vi "Set Syntax In Global.vi"(8 "error in":errorcluster, 10 "Syntax":T1, 11 "System no.":i32) -> (0 "error out":errorcluster)   [LabVIEW 2026]
uses:
  Syntax.ctl
  Global1.vi
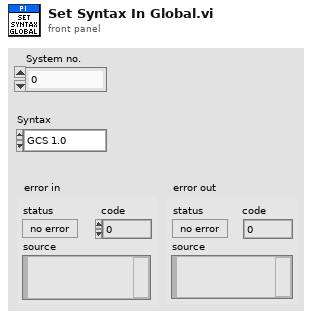
[diagram p1: front panel]
types:
  T1 = typedef "Syntax.ctl" = enum16{"GCS 1.0", "GCS 2.0", "GCS 3.0"}
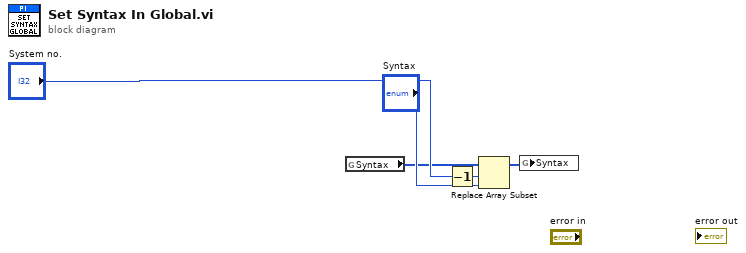
[diagram p0: block diagram]
diagram:
  n1 = global read "Global1.vi" "Syntax"() -> (w2:T1[])
  n2 = Decrement(x="System no.") -> (x-1=w5:i32)
  n3 = Replace Array Subset(array=w2, new element="Syntax", index=w5) -> (w1:T1[])
  n4 = global write "Global1.vi" "Syntax"(w1) -> ()
